vi "Get Relay Assignments.vi"(0 "VISA Session In":refnum<visa-resource-name>="OXYMAT", 1 "Target Address":u8=16 format="%.0x", 2 "Source Address":u8=208 format="%.0x", 7 "Option Board?":bool, 11 "error in (no error)":errorcluster) -> (4 "VISA Session Out":refnum<visa-resource-name>, 6 "Message Header":T2 {"Source Address" format="%.0x"; "Target Address" format="%.0x"}, 10 "Relay Assignments":T1(array[ring]), 13 "Success":bool, 15 "error out":errorcluster)   [LabVIEW 2019, in "Siemens ELAN.lvlib"]
doc: "Using the Siemens ELAN protocol, gets list of Autocal steps (as an array of enumerated values) from the addressed analyzer. Also returns a boolean indicating that the addressed device provided a valid response.\n\n$Revision:: 0 $\n$Modtime:: yy-mm-dd hh:mm $\n$Author:: Dboyd $"
uses:
  Siemens ELAN.lvlib
  Message Header.ctl
  Channel Status.ctl
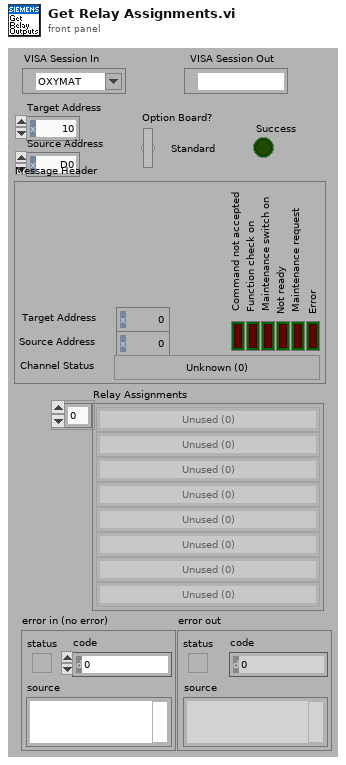
[diagram p1: front panel]
types:
  T1 = enum8{"Unused (0)", "Free", "Error", "Maintenance Request", "Calibration", "Component 1 Measuring Range 1 Selected", "Component 1 Measuring Range 2 Selected", "Component 1 Measuring Range 3 Selected", "Component 1 Measuring Range 4 Selected", "Component 1 Alarm 1 Triggered", "Component 1 Alarm 2 Triggered", "Function Check", "Valve for Sample Gas Open", "Valve for Zero Gas Open", "Valve for Cal Gas 1 Open", "Valve for Cal Gas 2 Open", "Valve for Cal Gas 3 Open", "Valve for Cal Gas 4 Open", "Measuring Point 1", "Measuring Point 2", "Measuring Point 3", "Measuring Point 4", "Measuring Point 5", "Measuring Point 6", "Signal from Measuring Point 1", "Signal from Measuring Point 2", "Signal from Measuring Point 3", "Signal from Measuring Point 4", "Signal from Measuring Point 5", "Signal from Measuring Point 6", "Signal Contact", "Reference Gas Flow", "Sample Gas Flow", "Valve for Zero Gas 2 Open", "Component 2 Measuring Range 1 Selected", "Component 2 Measuring Range 2 Selected", "Component 2 Measuring Range 3 Selected", "Component 2 Measuring Range 4 Selected", "Component 2 Limit 1 Triggered", "Component 2 Limit 2 Triggered", "Component 3 Measuring Range 2 Selected", "Component 3 Limit 1 Triggered", "Component 3 Limit 2 Triggered", "Component 4 Measuring Range 2 Selected", "Component 4 Limit 1 Triggered", "Component 4 Limit 2 Triggered", "Cal/Meas", "Unused (>46)"}[]
  T2 = typedef "Siemens ELAN.lvlib/Message Header.ctl" = cluster{"Target Address":u8, "Source Address":u8, "Error":bool, "Maintenance request":bool, "Not ready":bool, "Maintenance switch on":bool, "Function check on":bool, "Command not accepted":bool, "Channel Status":T3}
  T3 = typedef "Siemens ELAN.lvlib/Channel Status.ctl" = enum8{"Unknown (0)", "Warm-up", "Pause", "Standby", "Measure", "Zero calibration", "Adjust component slope", "Unknown (7)", "Adjust curve dip", "Adjust linearization sensitivity", "Adjust temperature compensation", "Adjust pressure compensation", "Adjust linearization zero", "Adjust flow sensor", "Autocal", "Adjust phase", "Zero calibration of O2 sensor", "Synchronous zero calibration", "Purging for synchronous zero calibration", "Adjust analog output", "Adjust analog input", "Cleaning", "Unknown (>21)"}
  T4 = enum8{"Unused (0)", "Free", "Error", "Maintenance Request", "Calibration", "Component 1 Measuring Range 1 Selected", "Component 1 Measuring Range 2 Selected", "Component 1 Measuring Range 3 Selected", "Component 1 Measuring Range 4 Selected", "Component 1 Alarm 1 Triggered", "Component 1 Alarm 2 Triggered", "Function Check", "Valve for Sample Gas Open", "Valve for Zero Gas Open", "Valve for Cal Gas 1 Open", "Valve for Cal Gas 2 Open", "Valve for Cal Gas 3 Open", "Valve for Cal Gas 4 Open", "Measuring Point 1", "Measuring Point 2", "Measuring Point 3", "Measuring Point 4", "Measuring Point 5", "Measuring Point 6", "Signal from Measuring Point 1", "Signal from Measuring Point 2", "Signal from Measuring Point 3", "Signal from Measuring Point 4", "Signal from Measuring Point 5", "Signal from Measuring Point 6", "Signal Contact", "Reference Gas Flow", "Sample Gas Flow", "Valve for Zero Gas 2 Open", "Component 2 Measuring Range 1 Selected", "Component 2 Measuring Range 2 Selected", "Component 2 Measuring Range 3 Selected", "Component 2 Measuring Range 4 Selected", "Component 2 Limit 1 Triggered", "Component 2 Limit 2 Triggered", "Component 3 Measuring Range 2 Selected", "Component 3 Limit 1 Triggered", "Component 3 Limit 2 Triggered", "Component 4 Measuring Range 2 Selected", "Component 4 Limit 1 Triggered", "Component 4 Limit 2 Triggered", "Cal/Meas", "Unused (>46)"}
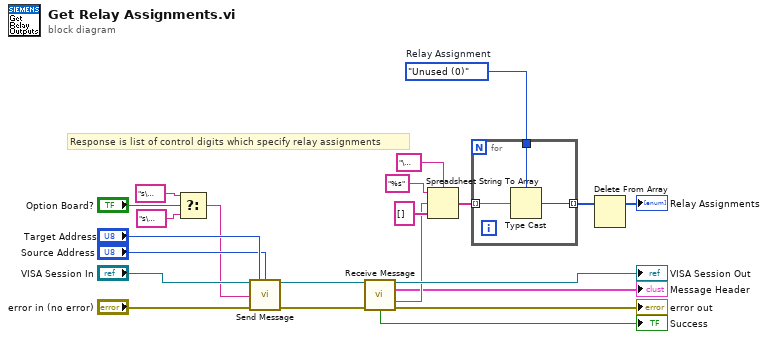
[diagram p0: block diagram]
diagram:
  w7 = T4."Unused (0)"  # Relay Assignment
  # "Response is list of control digits which specify relay assignments"
  n1 = Select(t="s\u0005" ("Command"), s="Option Board?", f="s\u0004" ("Command")) -> (s? t:f=w1:string)
  n2 = call "Send Message.vi"("VISA Session In"="VISA Session In", "Target Address"="Target Address", "Source Address"="Source Address", "Command"=w1, "error in (no error)"="error in (no error)") -> ("VISA Session Out"=w22:refnum<visa-resource-name>, "error out"=w21:errorcluster)  [unwired: 8 in, 1 out]
  n3 = call "Receive Message.vi"("VISA Session In"=w22, "error in (no error)"=w21) -> ("VISA Session Out"=→"VISA Session Out":refnum<visa-resource-name>, "Message Header"=→"Message Header":T2, "Response"=w12:string, "Success"=→"Success":bool, "error out"=→"error out":errorcluster)  [unwired: 8 in, 1 out]
  n4 = Spreadsheet String To Array(delimiter (Tab)="\u0000", format string="%s", spreadsheet string=w12, array type (2D Dbl)=string[] []) -> (array=w8:string[])
  n5 = for {
    tunnel: w8 -> [w25] mode=indexing
    tunnel: w7 -> [w24]
    tunnel: [w23] -> w6 mode=indexing
    n6 = Type Cast(type=w24, x=w25) -> (*(type *) &x=w23:T4)
  }
  n7 = Delete From Array(array=w6) -> (array with subset deleted=→"Relay Assignments":T1)  [unwired: 2 in, 1 out]
